vi "file get list from folder.vi"(8 "error in":errorcluster, 11 "path":path=path "C:/Documents and Settings/kubley.ONEPURDUE/Desktop/data analysis/modules/sequence calculation") -> (0 "error out":errorcluster, 3 "VI in folder":string[](array[string]))   [LabVIEW 2016]
doc: "takes vi's from a folder and displays them without the .vi"
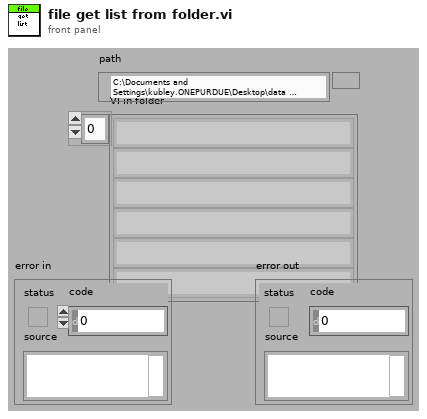
[diagram p1: front panel]
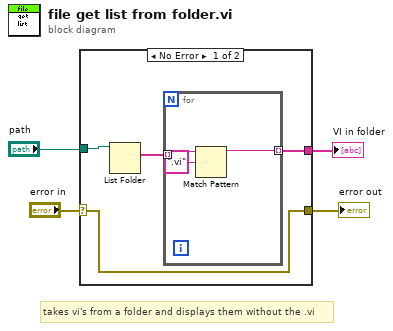
[diagram p0: block diagram]
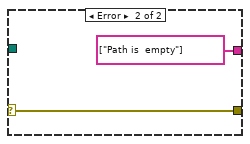
[diagram p2: hidden frame]
diagram:
  # "takes vi's from a folder and displays them without the .vi"
  n1 = case shown="No Error" "error in" {
    selector: "error in" -> [w5 w13]
    tunnel: "path" -> [w8 _]
    tunnel: [w6 string[] ["Path is  empty"]] -> w3
    tunnel: [w5 w13] -> w1
    frame No Error {
      n2 = List Folder(path=w8) -> (filenames=w7:string[])  [unwired: 3 in, 3 out]
      n3 = for {
        tunnel: w7 -> [w11] mode=indexing
        tunnel: [w9] -> w6 mode=indexing
        n4 = Match Pattern(string=w11, regular expression=".vi") -> (before substring=w9:string)  [unwired: 1 in, 3 out]
      }
    }
    frame Error {
    }
  }
  "VI in folder" <- w3
  "error out" <- w1
